vi "Driving-on-Line.vi"() -> ()   [LabVIEW 2016, in "EV3Group10.lvrbt"]
uses:
  EV3Group10.lvrbt
  <vilib>/NXT/Block Support/NXT_InputPort.ctl
  <vilib>/NXT/Block Support/NXT_OutputPort.ctl
  <vilib>/NXT/Dual Mode Library/Waits/Wait_Touch.vi
  <vilib>/NXT/Dual Mode Library/Display/drawText.vi
  <vilib>/NXT/Dual Mode Library/Waits/Wait_Num.vi
  <vilib>/NXT/Dual Mode Library/Sensors/EV3_Color_Reflect.vi
  <vilib>/NXT/NXTIO Xnodes/NXTIONodeSubVIs/NXTMoveMotors.vi
  <vilib>/NXT/NXTIO Xnodes/NXTIONodeSubVIs/NXTStopMotors.vi
  <vilib>/NXT/Dual Mode Library/Waits/Wait_LetGo.vi
  <vilib>/NXT/Dual Mode Library/Waits/Wait_Bump.vi
  <vilib>/NXT/NXTIO Xnodes/AddressXNode/NXTIOAddress.xnode
  <vilib>/NXT/NXTIO Xnodes/NXTIOXNode/NXTIO.xnode
  <vilib>/NXT/Subs/LVHSConnector.ctl
  <vilib>/NXT/LegoClasses/BrickReference/BrickReference.lvclass
panel:
  in  "Stopp":bool
  out "Signal 2":dbl
  out "Signal 1":dbl
  out "Average Signal":dbl
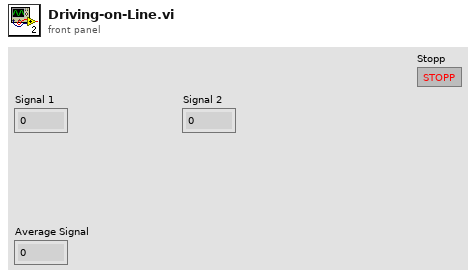
[diagram p1: front panel]
types:
  T1 = typedef "NXT_InputPort.ctl" = u32
  T2 = typedef "LVHSConnector.ctl" = refnum<class "BrickReference.lvclass">
  T3 = typedef "NXT_OutputPort.ctl" = u8
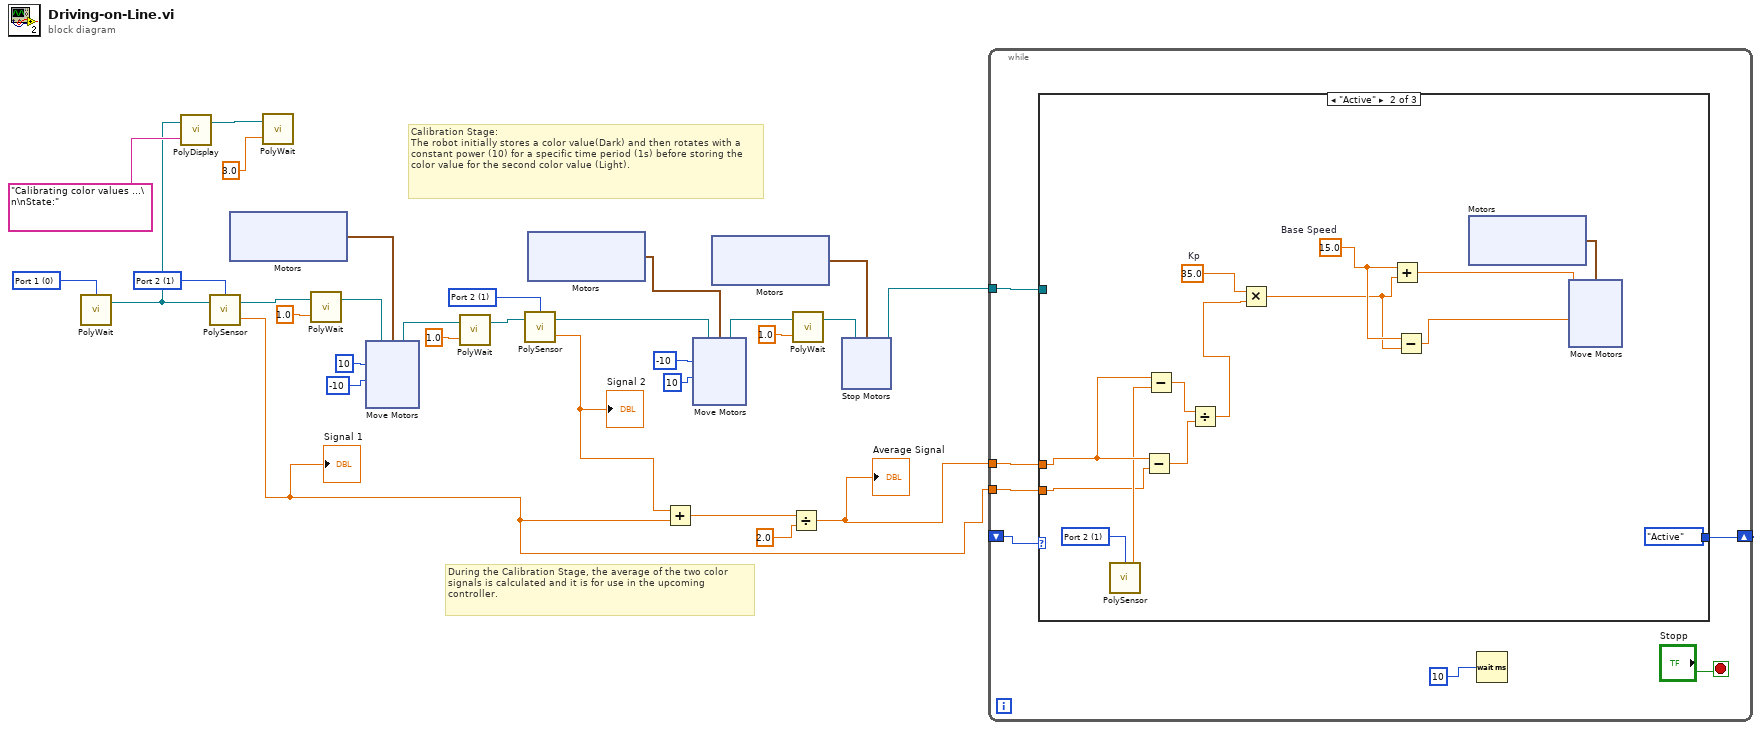
[diagram p0: block diagram]
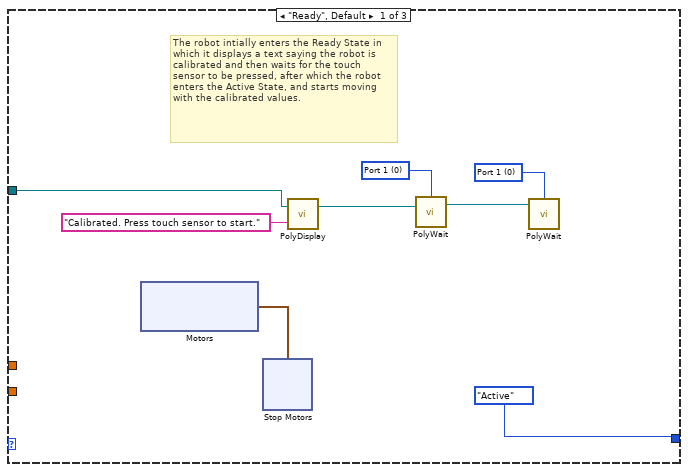
[diagram p2: hidden frame]
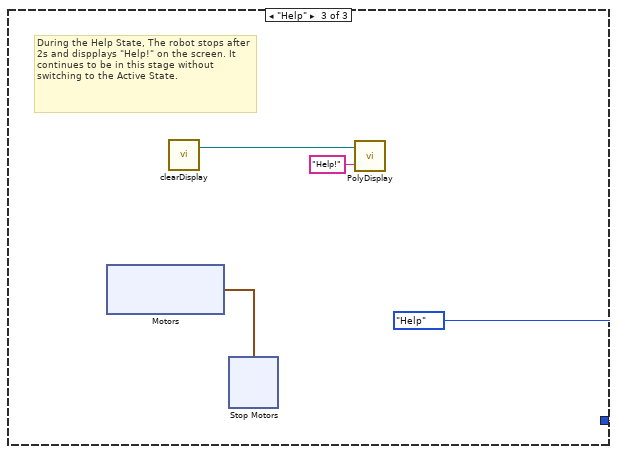
[diagram p3: hidden frame]
diagram:
  w11 = T1 1 items=["Port 1", "Port 2", "Port 3", "Port 4"] ("Port (Port 1)")
  w16 = T1 0 items=["Port 1", "Port 2", "Port 3", "Port 4"] ("Port (Port 1)")
  w30 = T1 1 items=["Port 1", "Port 2", "Port 3", "Port 4"] ("Port (Port 1)")
  # "During the Calibration Stage, the average of the two color signals is calculated and it is for use in the upcoming controller."
  # "Calibration Stage:\nThe robot initially stores a color value(Dark) and then rotates with a constant power (10) for a specific time period (1s) before storing the color value for the second color value (Light)."
  n1 = call-poly <vilib>:"PolyWait.vi"("Port (Port 1)"=w16) -> ("NXT/EV3"=w8:T2)  [unwired: 3 in]
  n2 = call-poly <vilib>:"PolyDisplay.vi"("Text"="Calibrating color values ...\n\nState:", "NXT/EV3"=w8) -> ("NXT/EV3"=w18:T2)  [unwired: 2 in]
  n3 = call-poly <vilib>:"PolySensor.vi"("NXT/EV3"=w8, "Port (Port 1)"=w11) -> ("Scaled Value"=w1:sgl, "NXT/EV3"=w10:T2)  [unwired: 1 in]
  "Signal 1" <- w1
  n4 = xnode "Motors"() -> ("Motor"=w29:cluster{"Port":T3, "Port":T3})
  n5 = call-poly <vilib>:"PolyWait.vi"("Time (1 sec)"=sgl 3.0, "NXT/EV3"=w18) -> ()  [unwired: 2 in, 1 out]
  n6 = call-poly <vilib>:"PolyWait.vi"("Time (1 sec)"=sgl 1.0, "NXT/EV3"=w10) -> ("NXT/EV3"=w12:T2)  [unwired: 2 in]
  n7 = xnode "Move Motors"("Power/Speed 2"=i8 -10, "Power/Speed 1"=i8 10, "Motors"=w29, "NXT/EV3"=w12) -> ("NXT/EV3"=w19:T2)
  n8 = call-poly <vilib>:"PolyWait.vi"("Time (1 sec)"=sgl 1.0, "NXT/EV3"=w19) -> ("NXT/EV3"=w15:T2)  [unwired: 2 in]
  n9 = call-poly <vilib>:"PolySensor.vi"("NXT/EV3"=w15, "Port (Port 1)"=w30) -> ("Scaled Value"=w4:sgl, "NXT/EV3"=w14:T2)  [unwired: 1 in]
  "Signal 2" <- w4
  n10 = xnode "Motors"() -> ("Motor"=w25:cluster{"Port":T3, "Port":T3})
  n11 = Add(x=w4, y=w1) -> (x+y=w7:sgl)
  n12 = xnode "Move Motors"("Power/Speed 2"=i8 10, "Power/Speed 1"=i8 -10, "Motors"=w25, "NXT/EV3"=w14) -> ("NXT/EV3"=w22:T2)
  n13 = xnode "Motors"() -> ("Motor"=w5:cluster{"Port":T3, "Port":T3})
  n14 = Divide(x=w7, y=sgl 2.0) -> (x/y=w2:sgl)
  "Average Signal" <- w2
  n15 = call-poly <vilib>:"PolyWait.vi"("Time (1 sec)"=sgl 1.0, "NXT/EV3"=w22) -> ("NXT/EV3"=w9:T2)  [unwired: 2 in]
  n16 = xnode "Stop Motors"("Motors"=w5, "NXT/EV3"=w9) -> ("NXT/EV3"=w3:T2)
  n17 = while {
    tunnel: w2 -> [w35]
    shift-right: [w31] -> _
    shift-left: _ -> [w33]
    tunnel: w3 -> [w36]
    tunnel: w1 -> [w32]
    stop <- "Stopp" stop-if-true
    n18 = case "Case-Struktur" shown="\"Active\"" w33 {
      tunnel: w36 -> [w44 _ _]
      tunnel: [enum16{"Ready", "Active", "Help", ""}."Active" enum16{"Ready", "Active", "Help", ""}."Active" enum16{"Ready", "Active", "Help", ""}."Help"] -> w31
      tunnel: w35 -> [_ w64 _]
      tunnel: w32 -> [_ w60 _]
      frame "Ready", Default {
        w40 = T1 0 items=["Port 1", "Port 2", "Port 3", "Port 4"] ("Port (Port 1)")
        w42 = T1 0 items=["Port 1", "Port 2", "Port 3", "Port 4"] ("Port (Port 1)")
        # "The robot intially enters the Ready State in which it displays a text saying the robot is calibrated and then waits for the touch sensor to be pressed, after which the robot enters the Active State, and starts moving with the calibrated values."
        n19 = xnode "Motors"() -> ("Motor"=w39:cluster{"Port":T3, "Port":T3})
        n20 = xnode "Stop Motors"("Motors"=w39) -> ()  [unwired: 1 in, 1 out]
        n21 = call-poly <vilib>:"PolyDisplay.vi"("Text"="Calibrated. Press touch sensor to start.", "NXT/EV3"=w44) -> ("NXT/EV3"=w43:T2)  [unwired: 2 in]
        n22 = call-poly <vilib>:"PolyWait.vi"("NXT/EV3"=w43, "Port (Port 1)"=w42) -> ("NXTEV3"=w41:T2)  [unwired: 2 in]
        n23 = call-poly <vilib>:"PolyWait.vi"("NXT/EV3"=w41, "Port (Port 1)"=w40) -> ()  [unwired: 2 in, 1 out]
      }
      frame "Active" {
        w62 = sgl 15.0  # Base Speed
        w63 = sgl 35.0  # Kp
        w65 = T1 1 items=["Port 1", "Port 2", "Port 3", "Port 4"] ("Port (Port 1)")
        n24 = call-poly <vilib>:"PolySensor.vi"("Port (Port 1)"=w65) -> ("Scaled Value"=w61:sgl)  [unwired: 2 in, 1 out]
        n25 = Subtract(x=w64, y=w60) -> (x-y=w58:sgl)
        n26 = Subtract(x=w64, y=w61) -> (x-y=w59:sgl)
        n27 = Divide(x=w59, y=w58) -> (x/y=w57:sgl)
        n28 = Multiply(x=w63, y=w57) -> (x*y=w53:sgl)
        n29 = Add(x=w62, y=w53) -> (x+y=w55:sgl)
        n30 = Subtract(x=w62, y=w53) -> (x-y=w54:sgl)
        n31 = xnode "Motors"() -> ("Motor"=w56:cluster{"Port":T3, "Port":T3})
        n32 = xnode "Move Motors"("Power/Speed 2"=w54, "Power/Speed 1"=w55, "Motors"=w56) -> ()  [unwired: 1 in, 1 out]
      }
      frame "Help" {
        # "During the Help State, The robot stops after 2s and dispplays \"Help!\" on the screen. It continues to be in this stage without switching to the Active State."
        n33 = xnode "Motors"() -> ("Motor"=w78:cluster{"Port":T3, "Port":T3})
        n34 = call <vilib>:"clearDisplay.vi"() -> ("NXT/EV3"=w77:T2)  [unwired: 4 in]
        n35 = xnode "Stop Motors"("Motors"=w78) -> ()  [unwired: 1 in, 1 out]
        n36 = call-poly <vilib>:"PolyDisplay.vi"("Text"="Help!", "NXT/EV3"=w77) -> ()  [unwired: 2 in, 1 out]
      }
    }
    n37 = Wait (ms)(milliseconds to wait=u32 10 ("Zu wartende ms")) -> ()  [unwired: 1 out]
  }
